vi "PhotodetectorTest.vi"(10 "loops x measure":i32=10, 11 "resource name":refnum<visa-resource-name>) -> (1 "Initialized PD":bool, 2 "Power":dbl format="%_7g", 3 "error out":errorcluster)   [LabVIEW 2018]
panel:
  out "Waveform Chart":dbl(graph)
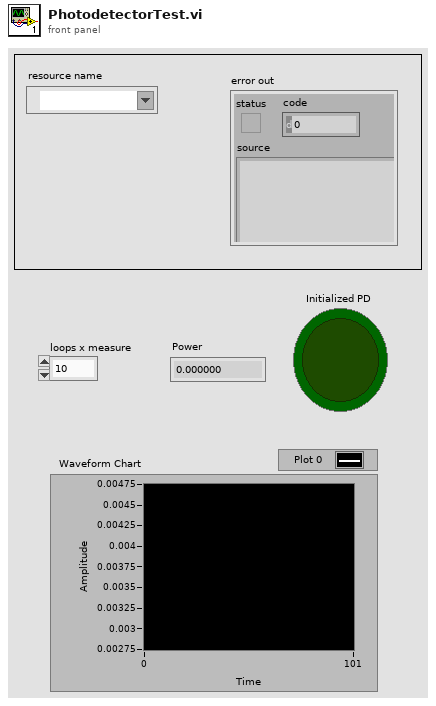
[diagram p1: front panel]
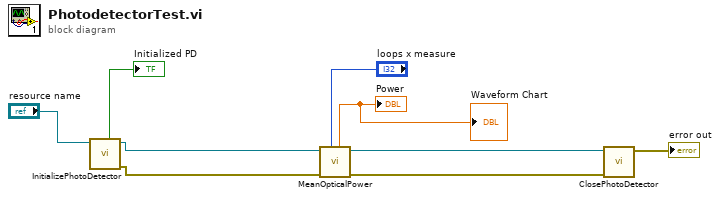
[diagram p0: block diagram]
diagram:
  n1 = call "InitializePhotoDetector.vi"("resource name"="resource name") -> ("error IO"=w1:errorcluster, "instrument handle out"=w6:refnum<visa-resource-name>, "Initialized PD"=→"Initialized PD":bool)  [unwired: 8 in]
  n2 = call "MeanOpticalPower.vi"("loops x measure"="loops x measure", "error out"=w1, "Visa Ref in"=w6) -> ("error out 2"=w4:errorcluster, "Visa ref out"=w5:refnum<visa-resource-name>, "Power"=→"Power" →"Waveform Chart":dbl)  [unwired: 6 in]
  n3 = call "ClosePhotoDetector.vi"("error in (no error)"=w4, "instrument handle"=w5) -> ("error out"=→"error out":errorcluster)  [unwired: 9 in]
